vi "specu1a 1.0.0 Read Status request.vi"(3 "error in (no error)":errorcluster, 5 "Device Handle":i32) -> (0 "error out":errorcluster, 1 "Status":T1, 2 "Device Handle out":i32)   [LabVIEW 2010]
uses:
  Controls/specu1a 1.0.0 Status.ctl
  WINDOWS/SYSTEM32/DRIVERS/specu1a.dll
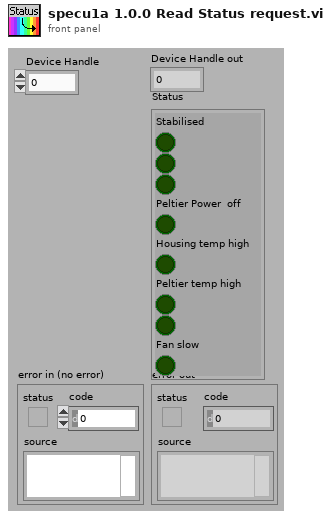
[diagram p1: front panel]
types:
  T1 = typedef "specu1a 1.0.0 Status.ctl" = cluster{"Stabilised":bool, bool, bool, "Peltier Power  off":bool, "Housing temp high":bool, "Peltier temp high":bool, bool, "Fan slow":bool}
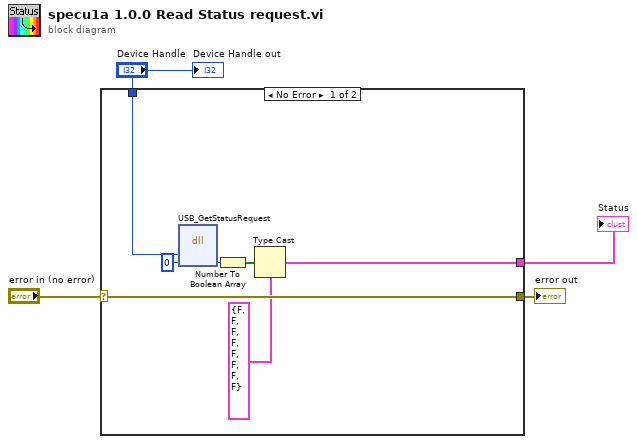
[diagram p0: block diagram]
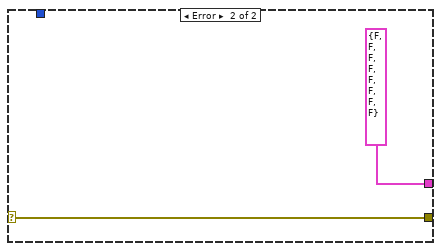
[diagram p2: hidden frame]
diagram:
  n1 = case shown="No Error" "error in (no error)" {
    selector: "error in (no error)" -> [w10 w13]
    tunnel: [w10 w13] -> w3
    tunnel: [w5 T1 {"Stabilised"=FALSE, FALSE, FALSE, "Peltier Power  off"=FALSE, "Housing temp high"=FALSE, "Peltier temp high"=FALSE, FALSE, "Fan slow"=FALSE} ("Status")] -> w1
    tunnel: "Device Handle" -> [w11 _]
    frame No Error {
      n2 = dll-call lib="C:/WINDOWS/SYSTEM32/DRIVERS/specu1a.dll" fn="USB_GetStatusRequest" label="1.0.0 Get Status request"("Device Handle"=w11, "Flag"=u8 0) -> ("Flag"=w8:u8)  [unwired: 5 in, 2 out]
      n3 = Number To Boolean Array(number=w8) -> (Boolean array=w7:bool[])
      n4 = Type Cast(type=T1 {"Stabilised"=FALSE, FALSE, FALSE, "Peltier Power  off"=FALSE, "Housing temp high"=FALSE, "Peltier temp high"=FALSE, FALSE, "Fan slow"=FALSE} ("Status"), x=w7) -> (*(type *) &x=w5:T1)
    }
    frame Error {
    }
  }
  "error out" <- w3
  "Status" <- w1
  "Device Handle out" <- "Device Handle"
